vi "Hide All Iteration Terminals.vi"(8 "error in (no error)":errorcluster, 11 "VI Refnum":refnum<vi>) -> (0 "error out":errorcluster, 3 "dup VI Refnum":refnum<vi>)   [LabVIEW 2023]
uses:
  <vilib>/Utility/traverseref.llb/TRef TravTarget.ctl
  <vilib>/Utility/traverseref.llb/VI Scripting - Traverse.lvlib
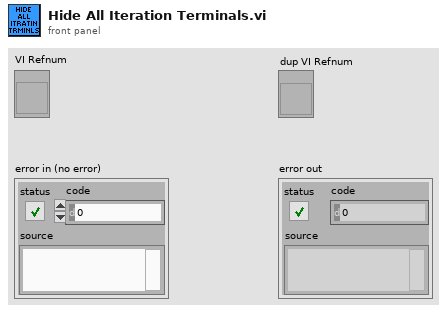
[diagram p1: front panel]
types:
  T1 = typedef "TRef TravTarget.ctl" = enum16{"FP", "BD", "Other"}
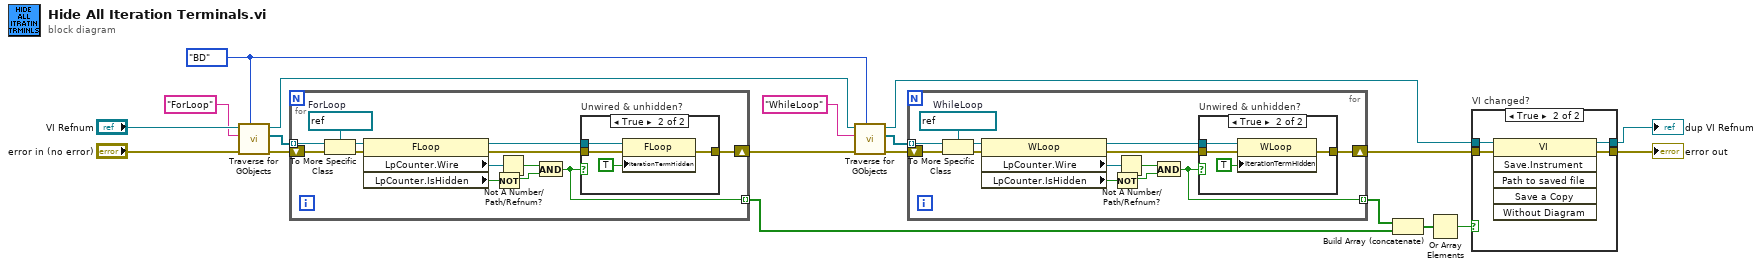
[diagram p0: block diagram]
diagram:
  w15 = TRef_TravTarget."BD" ("Traverse Target")
  n1 = call <vilib>:"Traverse for GObjects.vi"("Traverse Target"=w15, "error in (no error)"="error in (no error)", "Class Name"="ForLoop", "VI Refnum"="VI Refnum") -> ("error out"=w17:errorcluster, "References"=w19:refnum<vi>[], "dup VI Refnum"=w18:refnum<vi>)  [unwired: 4 in, 1 out]
  n2 = for {
    tunnel: w19 -> [w32] mode=indexing
    shift-right: [w24] -> w9
    shift-left: w17 -> [w27]
    tunnel: [w20] -> w4 mode=indexing
    w31 = refnum<vi> refnum  # ForLoop
    n3 = To More Specific Class(target class=w31, reference=w32, error in=w27) -> (specific class reference=w30:refnum<vi>, error out=w26:errorcluster)
    n4 = property class="FLoop"(reference=w30, error in=w26) -> (reference out=w29:refnum<vi>, error out=w25:errorcluster, "LpCounter.Wire"=w28:refnum<vi>, "LpCounter.IsHidden"=w23:bool)
    n5 = Not(x=w23) -> (.not. x?=w21:bool)
    n6 = Not A Number/Path/Refnum?(number/path/refnum=w28) -> (NaN/Path/Refnum?=w22:bool)
    n7 = And(x=w22, y=w21) -> (x .and. y?=w20:bool)
    n8 = case "Unwired & unhidden?" shown="True" w20 {
      tunnel: w29 -> [_ w36]
      tunnel: w25 -> [w33 w35]
      tunnel: [w33 w34] -> w24
      frame False {
      }
      frame True {
        n9 = property class="FLoop"(reference=w36, error in=w35, "IterationTermHidden"=TRUE ("Iteration Terminal Hidden?")) -> (error out=w34:errorcluster)  [unwired: 1 out]
      }
    }
  }
  n10 = call <vilib>:"Traverse for GObjects.vi"("Traverse Target"=w15, "error in (no error)"=w9, "Class Name"="WhileLoop", "VI Refnum"=w18) -> ("error out"=w8:errorcluster, "References"=w6:refnum<vi>[], "dup VI Refnum"=w5:refnum<vi>)  [unwired: 4 in, 1 out]
  n11 = for {
    shift-right: [w43] -> w7
    shift-left: w8 -> [w46]
    tunnel: [w39] -> w3 mode=indexing
    tunnel: w6 -> [w38] mode=indexing
    w50 = refnum<vi> refnum  # WhileLoop
    n12 = To More Specific Class(target class=w50, reference=w38, error in=w46) -> (specific class reference=w49:refnum<vi>, error out=w45:errorcluster)
    n13 = property class="WLoop"(reference=w49, error in=w45) -> (reference out=w48:refnum<vi>, error out=w44:errorcluster, "LpCounter.Wire"=w47:refnum<vi>, "LpCounter.IsHidden"=w42:bool)
    n14 = Not(x=w42) -> (.not. x?=w40:bool)
    n15 = Not A Number/Path/Refnum?(number/path/refnum=w47) -> (NaN/Path/Refnum?=w41:bool)
    n16 = And(x=w41, y=w40) -> (x .and. y?=w39:bool)
    n17 = case "Unwired & unhidden?" shown="True" w39 {
      tunnel: w48 -> [_ w54]
      tunnel: w44 -> [w51 w53]
      tunnel: [w51 w52] -> w43
      frame False {
      }
      frame True {
        n18 = property class="WLoop"(reference=w54, error in=w53, "IterationTermHidden"=TRUE ("Iteration Terminal Hidden?")) -> (error out=w52:errorcluster)  [unwired: 1 out]
      }
    }
  }
  n19 = Build Array (concatenate)(w3, w4) -> (w2:bool[])
  n20 = Or Array Elements(Boolean array=w2) -> (logical OR=w1:bool)
  n21 = case "VI changed?" shown="True" w1 {
    tunnel: [w56 w61] -> w13
    tunnel: [w57 w60] -> w12
    tunnel: w7 -> [w57 w59]
    tunnel: w5 -> [w56 w58]
    frame False {
    }
    frame True {
      n22 = invoke class="VI" method="Save.Instrument"(reference=w58, error in=w59) -> (reference out=w61:refnum<vi>, error out=w60:errorcluster)  [unwired: 4 in, 4 out]
    }
  }
  "error out" <- w12
  "dup VI Refnum" <- w13
